vi "Read Wavelength.vi"(8 "error in":errorcluster, 11 "LTB-1 in":refnum<class "LTB-1.lvclass">) -> (0 "error out":errorcluster, 2 "Wavelength (nm)":dbl, 3 "LTB-1 out":refnum<class "LTB-1.lvclass">)   [LabVIEW 2018, in "LTB-1.lvlib" / "LTB-1.lvclass"]
doc: "This is a parent VI that should be overidden by a child class. It will return the measured wavelength of the input signal.\n\nAuthor: Ron Dexter\nCompany: Luminar\nModified: 5/20/2018"
uses:
  LTB-1.lvclass
  C:/AME Test Engineering/LabVIEW/PPLs/EXFO/Parent/EXFO.lvlibp/EXFO.lvclass
  LTB-1.lvclass/LTB-1.ctl
  PPLs/EXFO/Parent/EXFO.lvlibp/Methods/Read Resource.vi
  3150 Driver/3150.lvlib
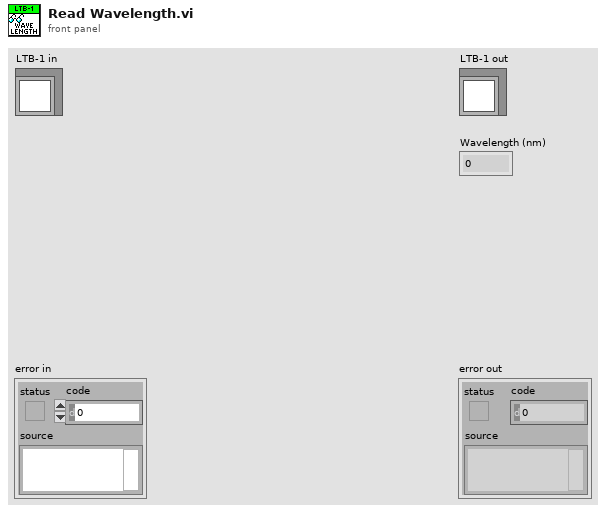
[diagram p1: front panel]
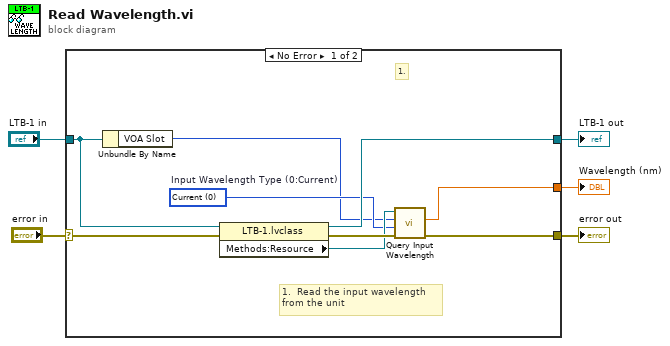
[diagram p0: block diagram]
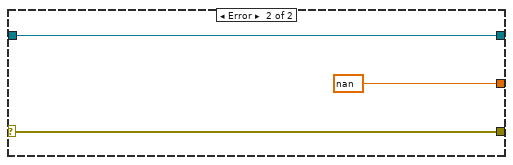
[diagram p2: hidden frame]
diagram:
  n1 = case shown="No Error" "error in" {
    selector: "error in" -> [w13 w17]
    tunnel: "LTB-1 in" -> [w12 w16]
    tunnel: [w11 w17] -> w4
    tunnel: [w8 nan ("Input Wavelength")] -> w3
    tunnel: [w14 w16] -> w2
    frame No Error {
      w7 = u16 0 items=["Current", "MINimum", "MAXimum", "DEFault"]  # Input Wavelength Type (0:Current)
      # "1.  Read the input wavelength \nfrom the unit"
      # "1."
      n2 = Unbundle By Name(w12) -> ("VOA Slot"=w6:i16)
      n3 = property class="LTB-1.lvclass"(reference=w12, error in=w13) -> (reference out=w14:refnum<class "LTB-1.lvclass">, error out=w10:errorcluster, "Methods:Resource"=w9:refnum<visa-resource-name>)
      n4 = call "Query Input Wavelength.vi"("error in (no error)"=w10, "Input Wavelength Type (0:Current)"=w7, "Platform Slot Number (10)"=w6, "VISA resource name"=w9) -> ("error out"=w11:errorcluster, "Input Wavelength"=w8:dbl)  [unwired: 5 in, 1 out]
    }
    frame Error {
    }
  }
  "error out" <- w4
  "LTB-1 out" <- w2
  "Wavelength (nm)" <- w3
